vi "Autonomous Independent.vi"   [LabVIEW 2011]
doc: "This VI is called when autonomous begins, and will automatically be terminated when autonomous ends. You can carry out timed or sensor driven robot movement independently without needing to return to the caller."
uses:
  Robot Global Data.vi
  System Set Points and States.vi
types:
  T1 = typedef "WPI_AnalogChannelDevRef.ctl" = cluster{"DevStatus":errorcluster, "Analog Module":T2, "Analog Channel":T3}
  T2 = typedef "FPGA_TypedefAnalogModule.ctl" = enum16{"Analog Module 1", "Analog Module 2"}
  T3 = typedef "FPGA_AIChannel.ctl" = enum8{"AI 1", "AI 2", "AI 3", "AI 4", "AI 5", "AI 6", "AI 7", "AI 8", "Invalid"}
  T4 = typedef "WPI_MotorControlDeviceRef.ctl" = cluster{"DeviceStatus":errorcluster, "Type":enum16{"PWM", "CAN"}, "PWM":cluster{"Digital Module":T5, "PWM Channel":T6, "DeadBand":T7}, "CAN":cluster{"Device Number":u8, "Control Mode":T8, "Semaphore":T9, "Max Vout":dbl}, "Invert":bool, "TransformRef":T10, "InvTransformRef":T10}
  T5 = typedef "FPGA_TypedefDigitalModule.ctl" = enum16{"Digital Module 1", "Digital Module 2"}
  T6 = typedef "FPGA_DIOPWMChannel.ctl" = enum8{"PWM 1", "PWM 2", "PWM 3", "PWM 4", "PWM 5", "PWM 6", "PWM 7", "PWM 8", "PWM 9", "PWM 10", "Invalid"}
  T7 = typedef "WPI_PWMDeadband.ctl" = cluster{"Name":string, "maxPositivePwm":i32, "minPositivePwm":i32, "centerPwm":i32, "maxNegativePwm":i32, "minNegativePwm":i32, "angularRange":u16}
  T8 = typedef "WPI_CANJaguar_ControlMode.ctl" = enum8{"Percent VBus", "Current", "Speed", "Position", "Voltage"}
  T9 = typedef "Semaphore RefNum" = refnum<k1>
  T10 = typedef "WPI_PWMTransform_ConPane.ctl" = refnum<vi>
  T11 = typedef "WPI_RobotDriveDevRef.ctl" = cluster{"DevStatus":errorcluster, "Motors[]":T4[], "Square Inputs":bool, "Max Output":dbl, "Isochronous":bool}
  T12 = typedef "WPI_DigitalInputDevRef.ctl" = cluster{"DevStatus":errorcluster, "DIO Channel":T13, "Digital Module":T5}
  T13 = typedef "FPGA_DIOChannel.ctl" = enum8{"DIO 1", "DIO 2", "DIO 3", "DIO 4", "DIO 5", "DIO 6", "DIO 7", "DIO 8", "DIO 9", "DIO 10", "DIO 11", "DIO 12", "DIO 13", "DIO 14", "Invalid"}
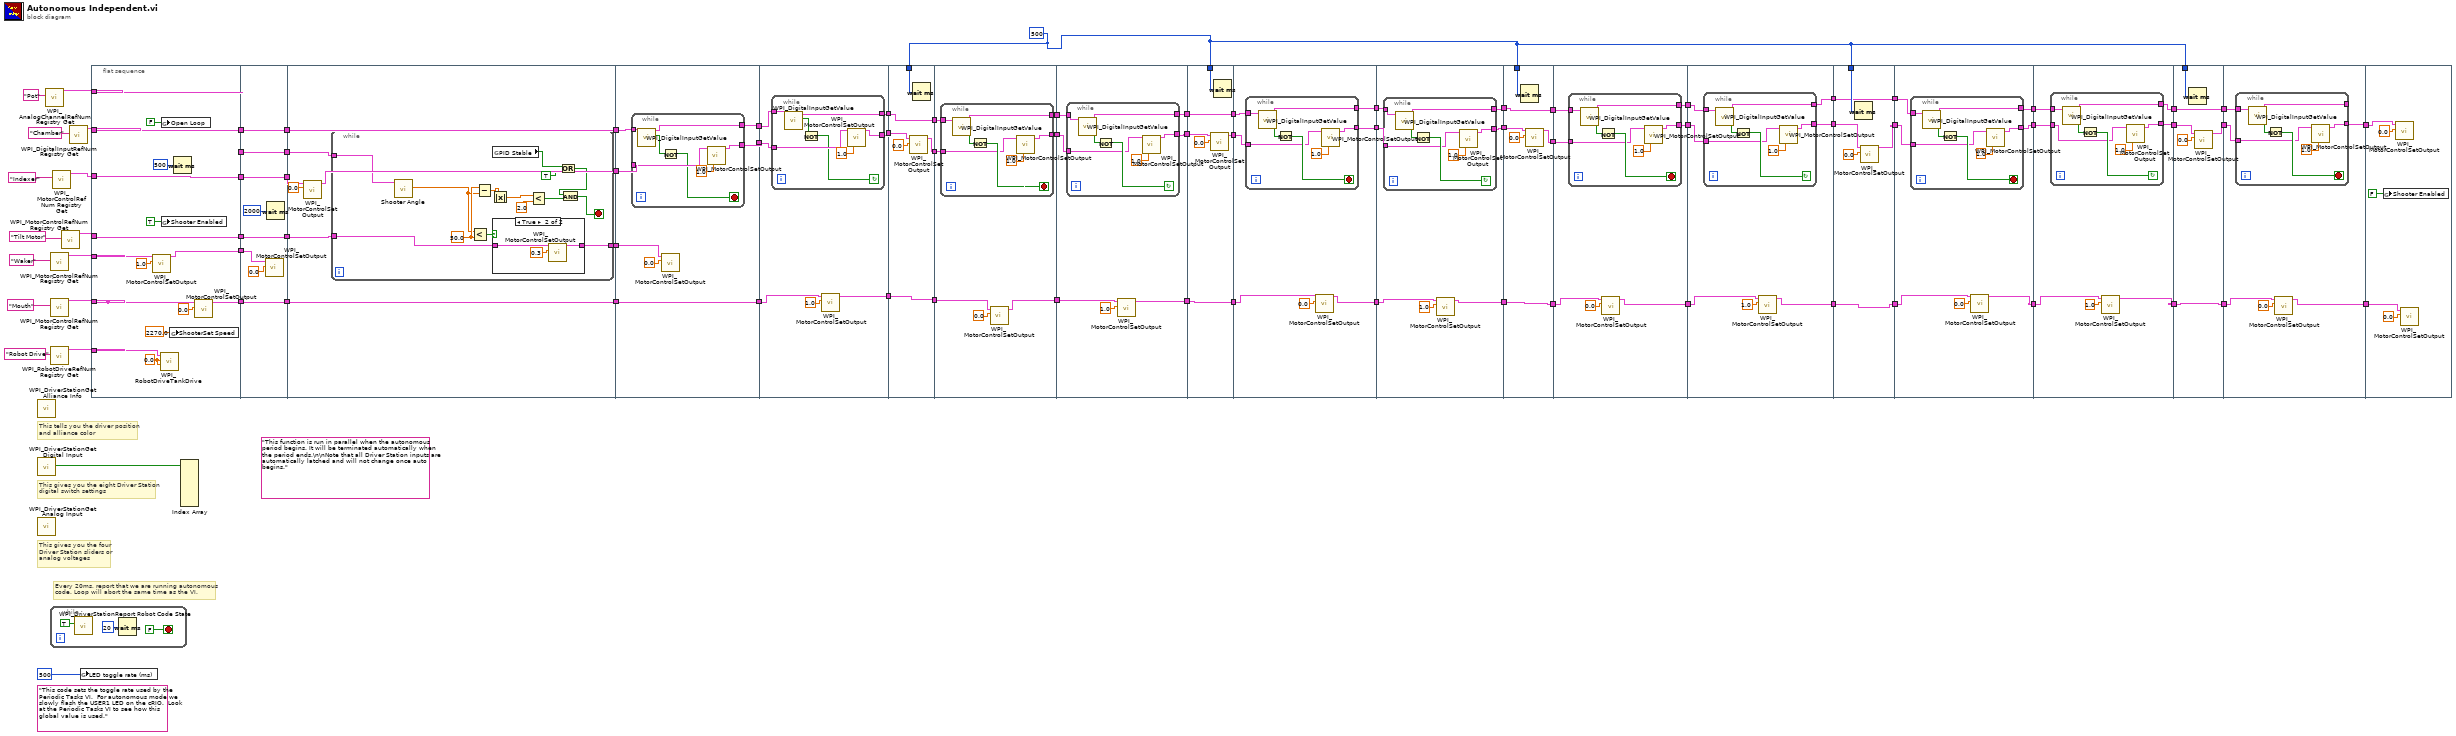
[diagram p0: block diagram]
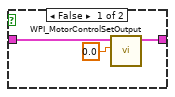
[diagram p2: hidden frame]
diagram:
  w7 = u32 500 ("milliseconds to wait")
  (unwired) "This code sets the toggle rate used by the Periodic Tasks VI.  For autonomous mode we slowly flash the USER1 LED on the cRIO.  Look at the Periodic Tasks VI to see how this global value is used."
  (unwired) "This function is run in parallel when the autonomous period begins. It will be terminated automatically when the period ends.\n\nNote that all Driver Station inputs are automatically latched and will not change once auto begins."
  # "Every 20ms, report that we are running autonomous\ncode. Loop will abort the same time as the VI."
  # "This tells you the driver position\nand alliance color"
  # "This gives you the eight Driver Station\ndigital switch settings"
  # "This gives you the four\nDriver Station sliders or\nanalog voltages"
  n1 = call <vilib>:"WPI_DriverStationGet Alliance Info.vi"() -> ()  [unwired: 12 out]
  n2 = call <vilib>:"WPI_DriverStationGet Digital Input.vi"() -> ("Driver Station Digital Input (1-8)"=w59:bool[])  [unwired: 11 out]
  n3 = call <vilib>:"WPI_DriverStationGet Analog Input.vi"() -> ()  [unwired: 12 out]
  n4 = call <vilib>:"WPI_AnalogChannelRefNum Registry Get.vi"("refnum name"="Pot") -> ("AIDeviceRef"=w67:T1)  [unwired: 9 in, 1 out]
  n5 = call <vilib>:"WPI_MotorControlRefNum Registry Get.vi"("refnum name"="Waker") -> ("MotorControlDevRef"=w63:T4)  [unwired: 9 in, 1 out]
  n6 = call <vilib>:"WPI_MotorControlRefNum Registry Get.vi"("refnum name"="Mouth") -> ("MotorControlDevRef"=w62:T4)  [unwired: 9 in, 1 out]
  n7 = call <vilib>:"WPI_RobotDriveRefNum Registry Get.vi"("refnum name"="Robot Drive") -> ("RobotDriveDevRef"=w60:T11)  [unwired: 9 in, 1 out]
  n8 = while {
    stop <- FALSE stop-if-true
    n9 = call <vilib>:"WPI_DriverStationReport Robot Code State.vi"("Autonomous"=TRUE) -> ()  [unwired: 10 in, 1 out]
    n10 = Wait (ms)(milliseconds to wait=u32 20) -> ()  [unwired: 1 out]
  }
  n11 = call <vilib>:"WPI_MotorControlRefNum Registry Get.vi"("refnum name"="Indexer") -> ("MotorControlDevRef"=w64:T4)  [unwired: 9 in, 1 out]
  n12 = call <vilib>:"WPI_MotorControlRefNum Registry Get.vi"("refnum name"="Tilt Motor") -> ("MotorControlDevRef"=w65:T4)  [unwired: 9 in, 1 out]
  n13 = call <vilib>:"WPI_DigitalInputRefNum Registry Get.vi"("refnum name"="Chamber") -> ("DigitalInputDevRef"=w71:T12)  [unwired: 9 in, 1 out]
  n14 = global write "Robot Global Data.vi" "LED toggle rate (ms)"(u32 500 ("LED ms toggle rate")) -> ()
  n15 = flat-sequence {
    tunnel: w64 -> [w93]
    tunnel: w63 -> [w91]
    tunnel: w71 -> [w92]
    tunnel: [w93] -> w32
    tunnel: [w92] -> w30
    tunnel: [w83] -> w28
    tunnel: [w86] -> _
    tunnel: [w89] -> w27
    tunnel: [w88] -> w25
    tunnel: w67 -> [w88]
    tunnel: [w87] -> w23
    tunnel: w65 -> [w87]
    tunnel: w62 -> [w86]
    tunnel: w60 -> [w85]
    tunnel: w32 -> [w106]
    tunnel: [w106] -> w31
    tunnel: w30 -> [w105]
    tunnel: [w105] -> w29
    tunnel: w28 -> [w99]
    tunnel: w27 -> [w104]
    tunnel: [w104] -> w26
    tunnel: w25 -> [w103]
    tunnel: [w103] -> w24
    tunnel: w23 -> [w102]
    tunnel: [w102] -> w22
    tunnel: w31 -> [w109]
    tunnel: [w107] -> w79
    tunnel: w29 -> [w114]
    tunnel: [w114] -> w78
    tunnel: [w113] -> w77
    tunnel: w26 -> [w113]
    tunnel: w24 -> [w112]
    tunnel: w22 -> [w111]
    tunnel: [w110] -> w66
    tunnel: w79 -> [w141]
    tunnel: w78 -> [w136]
    tunnel: [w138] -> w76
    tunnel: [w137] -> w75
    tunnel: w77 -> [w137]
    tunnel: w66 -> [w139]
    tunnel: [w135] -> w57
    tunnel: w76 -> [w155]
    tunnel: w75 -> [w150]
    tunnel: w57 -> [w154]
    tunnel: [w153] -> w54
    tunnel: [w152] -> w53
    tunnel: [w149] -> w52
    tunnel: [w163] -> w56
    tunnel: w54 -> [w165]
    tunnel: w53 -> [w167]
    tunnel: w52 -> [w163]
    tunnel: [w166] -> w51
    tunnel: [w165] -> w48
    tunnel: w7 -> [w164]
    tunnel: w56 -> [w170]
    tunnel: [w169] -> w55
    tunnel: w51 -> [w175]
    tunnel: [w174] -> w50
    tunnel: [w173] -> w49
    tunnel: w48 -> [w172]
    tunnel: w55 -> [w188]
    tunnel: w50 -> [w187]
    tunnel: w49 -> [w186]
    tunnel: [w185] -> w47
    tunnel: [w184] -> w45
    tunnel: [w183] -> w43
    tunnel: w47 -> [w201]
    tunnel: [w200] -> w46
    tunnel: w45 -> [w200]
    tunnel: [w199] -> w44
    tunnel: w43 -> [w197]
    tunnel: [w197] -> w42
    tunnel: w7 -> [w198]
    tunnel: w46 -> [w208]
    tunnel: w44 -> [w209]
    tunnel: w42 -> [w204]
    tunnel: [w203] -> w41
    tunnel: [w207] -> w40
    tunnel: [w206] -> w39
    tunnel: w41 -> [w218]
    tunnel: w40 -> [w223]
    tunnel: w39 -> [w222]
    tunnel: [w217] -> w38
    tunnel: [w221] -> w37
    tunnel: [w220] -> w36
    tunnel: w38 -> [w231]
    tunnel: w37 -> [w233]
    tunnel: w36 -> [w235]
    tunnel: w7 -> [w234]
    tunnel: [w233] -> w35
    tunnel: [w232] -> w34
    tunnel: [w231] -> w33
    tunnel: w35 -> [w243]
    tunnel: w34 -> [w242]
    tunnel: [w237] -> w19
    tunnel: w33 -> [w238]
    tunnel: [w241] -> w17
    tunnel: [w240] -> w16
    tunnel: w19 -> [w252]
    tunnel: [w251] -> w18
    tunnel: w17 -> [w257]
    tunnel: w16 -> [w256]
    tunnel: [w255] -> w15
    tunnel: [w254] -> w14
    tunnel: w18 -> [w265]
    tunnel: [w265] -> w21
    tunnel: [w268] -> w20
    tunnel: w15 -> [w269]
    tunnel: w7 -> [w267]
    tunnel: w14 -> [w266]
    tunnel: [w266] -> w13
    tunnel: w21 -> [w272]
    tunnel: [w271] -> w12
    tunnel: w20 -> [w277]
    tunnel: [w275] -> w11
    tunnel: w13 -> [w276]
    tunnel: [w274] -> w10
    tunnel: w12 -> [w286]
    tunnel: [w285] -> w9
    tunnel: w11 -> [w291]
    tunnel: [w289] -> w8
    tunnel: w10 -> [w290]
    tunnel: [w288] -> w2
    tunnel: w9 -> [w299]
    tunnel: [w299] -> w6
    tunnel: w8 -> [w302]
    tunnel: [w303] -> w4
    tunnel: w7 -> [w301]
    tunnel: w2 -> [w300]
    tunnel: [w300] -> w1
    tunnel: w6 -> [w306]
    tunnel: [w305] -> w5
    tunnel: w4 -> [w309]
    tunnel: [w310] -> w3
    tunnel: w1 -> [w308]
    tunnel: w5 -> [w320]
    tunnel: w3 -> [w318]
    frame #0 {
      w84 = 0.0 ("Left axis value")
      n16 = call <vilib>:"WPI_MotorControlSetOutput.vi"("Output"=1.0, "MotorControlDevRef"=w91) -> ("MotorControlDevRef"=w83:T4)  [unwired: 8 in, 1 out]
      n17 = call <vilib>:"WPI_RobotDriveTankDrive.vi"("Right axis value"=w84, "Left axis value"=w84, "RobotDriveDevRef"=w85) -> ()  [unwired: 7 in, 2 out]
      n18 = global write "System Set Points and States.vi" "Open Loop"(FALSE ("Open Loop")) -> ()
      n19 = global write "System Set Points and States.vi" "Shooter Enabled"(TRUE ("Shooter Enabled")) -> ()
      n20 = global write "System Set Points and States.vi" "ShooterSet Speed"(2270.0) -> ()
      n21 = Wait (ms)(milliseconds to wait=u32 500) -> ()  [unwired: 1 out]
      n22 = call <vilib>:"WPI_MotorControlSetOutput.vi"("Output"=0.0, "MotorControlDevRef"=w86) -> ("MotorControlDevRef"=w89:T4)  [unwired: 8 in, 1 out]
    }
    frame #1 {
      n23 = call <vilib>:"WPI_MotorControlSetOutput.vi"("Output"=0.0, "MotorControlDevRef"=w99) -> ()  [unwired: 8 in, 2 out]
      n24 = Wait (ms)(milliseconds to wait=u32 2000) -> ()  [unwired: 1 out]
    }
    frame #2 {
      n25 = call <vilib>:"WPI_MotorControlSetOutput.vi"("Output"=0.0, "MotorControlDevRef"=w109) -> ("MotorControlDevRef"=w107:T4)  [unwired: 8 in, 1 out]
      n26 = while {
        tunnel: w111 -> [w128]
        tunnel: w112 -> [w116]
        tunnel: [w122] -> w110
        stop <- w121 stop-if-true
        w123 = 50.0 ("y")
        n27 = call "Shooter Angle.vi"("AIDeviceRef"=w116) -> ("Shoter Angle"=w115:dbl)  [unwired: 9 in, 1 out]
        n28 = Less?(x=w115, y=w123) -> (x < y?=w127:bool)
        n29 = Subtract(x=w123, y=w115) -> (x-y=w126:dbl)
        n30 = Absolute Value(x=w126) -> (abs(x)=w125:dbl)
        n31 = case shown="True" w127 {
          tunnel: w128 -> [w130 w133]
          tunnel: [w129 w132] -> w122
          frame False {
            n32 = call <vilib>:"WPI_MotorControlSetOutput.vi"("Output"=0.0, "MotorControlDevRef"=w130) -> ("MotorControlDevRef"=w129:T4)  [unwired: 8 in, 1 out]
          }
          frame True {
            n33 = call <vilib>:"WPI_MotorControlSetOutput.vi"("Output"=0.3, "MotorControlDevRef"=w133) -> ("MotorControlDevRef"=w132:T4)  [unwired: 8 in, 1 out]
          }
        }
        n34 = global read "System Set Points and States.vi" "PID Stable"() -> (w119:bool)
        n35 = Less?(x=w125, y=2.0) -> (x < y?=w120:bool)
        n36 = Or(x=w119, y=TRUE) -> (x .or. y?=w118:bool)
        n37 = And(x=w118, y=w120) -> (x .and. y?=w121:bool)
      }
    }
    frame #3 {
      n38 = while {
        tunnel: w141 -> [w148]
        tunnel: [w147] -> w138
        tunnel: w136 -> [w144]
        tunnel: [w142] -> w135
        stop <- w143 stop-if-true
        n39 = call <vilib>:"WPI_DigitalInputGetValue.vi"("DigitalInputDevRef"=w144) -> ("Value"=w145:bool, "DigitalInputDevRef"=w142:T12)  [unwired: 8 in, 1 out]
        n40 = Not(x=w145) -> (.not. x?=w143:bool)
        n41 = call <vilib>:"WPI_MotorControlSetOutput.vi"("Output"=1.0, "MotorControlDevRef"=w148) -> ("MotorControlDevRef"=w147:T4)  [unwired: 8 in, 1 out]
      }
      n42 = call <vilib>:"WPI_MotorControlSetOutput.vi"("Output"=0.0, "MotorControlDevRef"=w139) -> ()  [unwired: 8 in, 2 out]
    }
    frame #4 {
      n43 = while {
        tunnel: w155 -> [w162]
        tunnel: [w161] -> w152
        tunnel: w154 -> [w158]
        tunnel: [w156] -> w153
        stop <- w157 continue-if-true
        n44 = call <vilib>:"WPI_DigitalInputGetValue.vi"("DigitalInputDevRef"=w158) -> ("Value"=w159:bool, "DigitalInputDevRef"=w156:T12)  [unwired: 8 in, 1 out]
        n45 = Not(x=w159) -> (.not. x?=w157:bool)
        n46 = call <vilib>:"WPI_MotorControlSetOutput.vi"("Output"=1.0, "MotorControlDevRef"=w162) -> ("MotorControlDevRef"=w161:T4)  [unwired: 8 in, 1 out]
      }
      n47 = call <vilib>:"WPI_MotorControlSetOutput.vi"("Output"=1.0, "MotorControlDevRef"=w150) -> ("MotorControlDevRef"=w149:T4)  [unwired: 8 in, 1 out]
    }
    frame #5 {
      n48 = call <vilib>:"WPI_MotorControlSetOutput.vi"("Output"=0.0, "MotorControlDevRef"=w167) -> ("MotorControlDevRef"=w166:T4)  [unwired: 8 in, 1 out]
      n49 = Wait (ms)(milliseconds to wait=w164) -> ()  [unwired: 1 out]
    }
    frame #6 {
      n50 = while {
        tunnel: [w182] -> w173
        tunnel: [w178] -> w174
        tunnel: w175 -> [w177]
        tunnel: w172 -> [w176]
        stop <- w179 stop-if-true
        n51 = call <vilib>:"WPI_DigitalInputGetValue.vi"("DigitalInputDevRef"=w176) -> ("Value"=w180:bool, "DigitalInputDevRef"=w178:T12)  [unwired: 8 in, 1 out]
        n52 = Not(x=w180) -> (.not. x?=w179:bool)
        n53 = call <vilib>:"WPI_MotorControlSetOutput.vi"("Output"=1.0, "MotorControlDevRef"=w177) -> ("MotorControlDevRef"=w182:T4)  [unwired: 8 in, 1 out]
      }
      n54 = call <vilib>:"WPI_MotorControlSetOutput.vi"("Output"=0.0, "MotorControlDevRef"=w170) -> ("MotorControlDevRef"=w169:T4)  [unwired: 8 in, 1 out]
    }
    frame #7 {
      n55 = while {
        tunnel: [w196] -> w185
        tunnel: [w192] -> w184
        tunnel: w186 -> [w191]
        tunnel: w187 -> [w190]
        stop <- w193 continue-if-true
        n56 = call <vilib>:"WPI_DigitalInputGetValue.vi"("DigitalInputDevRef"=w190) -> ("Value"=w194:bool, "DigitalInputDevRef"=w192:T12)  [unwired: 8 in, 1 out]
        n57 = Not(x=w194) -> (.not. x?=w193:bool)
        n58 = call <vilib>:"WPI_MotorControlSetOutput.vi"("Output"=1.0, "MotorControlDevRef"=w191) -> ("MotorControlDevRef"=w196:T4)  [unwired: 8 in, 1 out]
      }
      n59 = call <vilib>:"WPI_MotorControlSetOutput.vi"("Output"=1.0, "MotorControlDevRef"=w188) -> ("MotorControlDevRef"=w183:T4)  [unwired: 8 in, 1 out]
    }
    frame #8 {
      n60 = call <vilib>:"WPI_MotorControlSetOutput.vi"("Output"=0.0, "MotorControlDevRef"=w201) -> ("MotorControlDevRef"=w199:T4)  [unwired: 8 in, 1 out]
      n61 = Wait (ms)(milliseconds to wait=w198) -> ()  [unwired: 1 out]
    }
    frame #9 {
      n62 = while {
        tunnel: [w216] -> w206
        tunnel: [w212] -> w207
        tunnel: w209 -> [w211]
        tunnel: w208 -> [w210]
        stop <- w213 stop-if-true
        n63 = call <vilib>:"WPI_DigitalInputGetValue.vi"("DigitalInputDevRef"=w210) -> ("Value"=w214:bool, "DigitalInputDevRef"=w212:T12)  [unwired: 8 in, 1 out]
        n64 = Not(x=w214) -> (.not. x?=w213:bool)
        n65 = call <vilib>:"WPI_MotorControlSetOutput.vi"("Output"=1.0, "MotorControlDevRef"=w211) -> ("MotorControlDevRef"=w216:T4)  [unwired: 8 in, 1 out]
      }
      n66 = call <vilib>:"WPI_MotorControlSetOutput.vi"("Output"=0.0, "MotorControlDevRef"=w204) -> ("MotorControlDevRef"=w203:T4)  [unwired: 8 in, 1 out]
    }
    frame #10 {
      n67 = while {
        tunnel: [w230] -> w220
        tunnel: [w226] -> w221
        tunnel: w222 -> [w225]
        tunnel: w223 -> [w224]
        stop <- w227 continue-if-true
        n68 = call <vilib>:"WPI_DigitalInputGetValue.vi"("DigitalInputDevRef"=w224) -> ("Value"=w228:bool, "DigitalInputDevRef"=w226:T12)  [unwired: 8 in, 1 out]
        n69 = Not(x=w228) -> (.not. x?=w227:bool)
        n70 = call <vilib>:"WPI_MotorControlSetOutput.vi"("Output"=1.0, "MotorControlDevRef"=w225) -> ("MotorControlDevRef"=w230:T4)  [unwired: 8 in, 1 out]
      }
      n71 = call <vilib>:"WPI_MotorControlSetOutput.vi"("Output"=1.0, "MotorControlDevRef"=w218) -> ("MotorControlDevRef"=w217:T4)  [unwired: 8 in, 1 out]
    }
    frame #11 {
      n72 = Wait (ms)(milliseconds to wait=w234) -> ()  [unwired: 1 out]
      n73 = call <vilib>:"WPI_MotorControlSetOutput.vi"("Output"=0.0, "MotorControlDevRef"=w235) -> ("MotorControlDevRef"=w232:T4)  [unwired: 8 in, 1 out]
    }
    frame #12 {
      n74 = while {
        tunnel: [w250] -> w241
        tunnel: [w246] -> w240
        tunnel: w242 -> [w245]
        tunnel: w243 -> [w244]
        stop <- w247 stop-if-true
        n75 = call <vilib>:"WPI_DigitalInputGetValue.vi"("DigitalInputDevRef"=w244) -> ("Value"=w248:bool, "DigitalInputDevRef"=w246:T12)  [unwired: 8 in, 1 out]
        n76 = Not(x=w248) -> (.not. x?=w247:bool)
        n77 = call <vilib>:"WPI_MotorControlSetOutput.vi"("Output"=1.0, "MotorControlDevRef"=w245) -> ("MotorControlDevRef"=w250:T4)  [unwired: 8 in, 1 out]
      }
      n78 = call <vilib>:"WPI_MotorControlSetOutput.vi"("Output"=0.0, "MotorControlDevRef"=w238) -> ("MotorControlDevRef"=w237:T4)  [unwired: 8 in, 1 out]
    }
    frame #13 {
      n79 = while {
        tunnel: [w264] -> w255
        tunnel: [w260] -> w254
        tunnel: w257 -> [w259]
        tunnel: w256 -> [w258]
        stop <- w261 continue-if-true
        n80 = call <vilib>:"WPI_DigitalInputGetValue.vi"("DigitalInputDevRef"=w258) -> ("Value"=w262:bool, "DigitalInputDevRef"=w260:T12)  [unwired: 8 in, 1 out]
        n81 = Not(x=w262) -> (.not. x?=w261:bool)
        n82 = call <vilib>:"WPI_MotorControlSetOutput.vi"("Output"=1.0, "MotorControlDevRef"=w259) -> ("MotorControlDevRef"=w264:T4)  [unwired: 8 in, 1 out]
      }
      n83 = call <vilib>:"WPI_MotorControlSetOutput.vi"("Output"=1.0, "MotorControlDevRef"=w252) -> ("MotorControlDevRef"=w251:T4)  [unwired: 8 in, 1 out]
    }
    frame #14 {
      n84 = Wait (ms)(milliseconds to wait=w267) -> ()  [unwired: 1 out]
      n85 = call <vilib>:"WPI_MotorControlSetOutput.vi"("Output"=0.0, "MotorControlDevRef"=w269) -> ("MotorControlDevRef"=w268:T4)  [unwired: 8 in, 1 out]
    }
    frame #15 {
      n86 = while {
        tunnel: [w284] -> w275
        tunnel: [w280] -> w274
        tunnel: w277 -> [w279]
        tunnel: w276 -> [w278]
        stop <- w281 stop-if-true
        n87 = call <vilib>:"WPI_DigitalInputGetValue.vi"("DigitalInputDevRef"=w278) -> ("Value"=w282:bool, "DigitalInputDevRef"=w280:T12)  [unwired: 8 in, 1 out]
        n88 = Not(x=w282) -> (.not. x?=w281:bool)
        n89 = call <vilib>:"WPI_MotorControlSetOutput.vi"("Output"=1.0, "MotorControlDevRef"=w279) -> ("MotorControlDevRef"=w284:T4)  [unwired: 8 in, 1 out]
      }
      n90 = call <vilib>:"WPI_MotorControlSetOutput.vi"("Output"=0.0, "MotorControlDevRef"=w272) -> ("MotorControlDevRef"=w271:T4)  [unwired: 8 in, 1 out]
    }
    frame #16 {
      n91 = while {
        tunnel: [w298] -> w289
        tunnel: [w294] -> w288
        tunnel: w290 -> [w293]
        tunnel: w291 -> [w292]
        stop <- w295 continue-if-true
        n92 = call <vilib>:"WPI_DigitalInputGetValue.vi"("DigitalInputDevRef"=w293) -> ("Value"=w296:bool, "DigitalInputDevRef"=w294:T12)  [unwired: 8 in, 1 out]
        n93 = Not(x=w296) -> (.not. x?=w295:bool)
        n94 = call <vilib>:"WPI_MotorControlSetOutput.vi"("Output"=1.0, "MotorControlDevRef"=w292) -> ("MotorControlDevRef"=w298:T4)  [unwired: 8 in, 1 out]
      }
      n95 = call <vilib>:"WPI_MotorControlSetOutput.vi"("Output"=1.0, "MotorControlDevRef"=w286) -> ("MotorControlDevRef"=w285:T4)  [unwired: 8 in, 1 out]
    }
    frame #17 {
      n96 = Wait (ms)(milliseconds to wait=w301) -> ()  [unwired: 1 out]
      n97 = call <vilib>:"WPI_MotorControlSetOutput.vi"("Output"=0.0, "MotorControlDevRef"=w302) -> ("MotorControlDevRef"=w303:T4)  [unwired: 8 in, 1 out]
    }
    frame #18 {
      n98 = while {
        tunnel: [w317] -> w310
        tunnel: [w313] -> _
        tunnel: w309 -> [w312]
        tunnel: w308 -> [w311]
        stop <- w314 stop-if-true
        n99 = call <vilib>:"WPI_DigitalInputGetValue.vi"("DigitalInputDevRef"=w311) -> ("Value"=w315:bool, "DigitalInputDevRef"=w313:T12)  [unwired: 8 in, 1 out]
        n100 = Not(x=w315) -> (.not. x?=w314:bool)
        n101 = call <vilib>:"WPI_MotorControlSetOutput.vi"("Output"=1.0, "MotorControlDevRef"=w312) -> ("MotorControlDevRef"=w317:T4)  [unwired: 8 in, 1 out]
      }
      n102 = call <vilib>:"WPI_MotorControlSetOutput.vi"("Output"=0.0, "MotorControlDevRef"=w306) -> ("MotorControlDevRef"=w305:T4)  [unwired: 8 in, 1 out]
    }
    frame #19 {
      n103 = global write "System Set Points and States.vi" "Shooter Enabled"(FALSE ("Shooter Enabled")) -> ()
      n104 = call <vilib>:"WPI_MotorControlSetOutput.vi"("Output"=0.0, "MotorControlDevRef"=w318) -> ()  [unwired: 8 in, 2 out]
      n105 = call <vilib>:"WPI_MotorControlSetOutput.vi"("Output"=0.0, "MotorControlDevRef"=w320) -> ()  [unwired: 8 in, 2 out]
    }
  }
  n106 = Index Array(array=w59) -> ()  [unwired: 8 in, 8 out]
